vi "SL Basic Interface.vi"() -> ()   [LabVIEW 2016]
uses:
  source code/LSL components/scripts/scripts manager/scripts manager.lvclass
  source code/LSL components/output terminal/SystemLink OT/SystemLinkOutputTerminal.lvclass
  E:/Repository/LabVIEW Script Language/source code/LSL components/output terminal/Plain OT/PainOutputTerminal.lvclass
  E:/Repository/LabVIEW Script Language/source code/LSL components/output terminal/Base/Output Terminal.lvclass
  source code/LSL components/output terminal/Plain OT/PainOutputTerminal.lvclass/PainOutputTerminal.ctl
  source code/LSL components/output terminal/SystemLink OT/SystemLinkOutputTerminal.lvclass/SystemLinkOutputTerminal.ctl
  source code/LSL components/variables/RT Variables/RT Variables.lvclass
  source code/LSL components/scripts/scripts manager/scripts manager.lvclass/scripts manager.ctl
  <vilib>/Skyline/Message/AMQP/NI Skyline Message AMQP (Async).lvclass
  source code/LSL components/output terminal/Plain OT/properties/Write Output Terminal.vi
  source code/LSL components/output terminal/SystemLink OT/properties/Write SL async ref.vi
  source code/LSL components/output terminal/SystemLink OT/properties/Write Publish Topic.vi
  source code/LSL components/scripts/scripts manager/properties/Write Scripts.vi
  <vilib>/Skyline/Message/AMQP/async/Open (Async).vi
  <vilib>/Skyline/Utilities/NI Skyline Utilities.lvlib
  <vilib>/Skyline/Message/NI Skyline Message.lvclass
panel:
  in  "Help":bool
  in  "Script Compile":bool
  in  "Script Save":bool
  in  "Script Delete":bool
  in  "Script New":bool
  in  "Script Run":bool
  in  "Script Files":i32(listbox)
  out "Output Terminal":string
  in  "scripting pane":T1
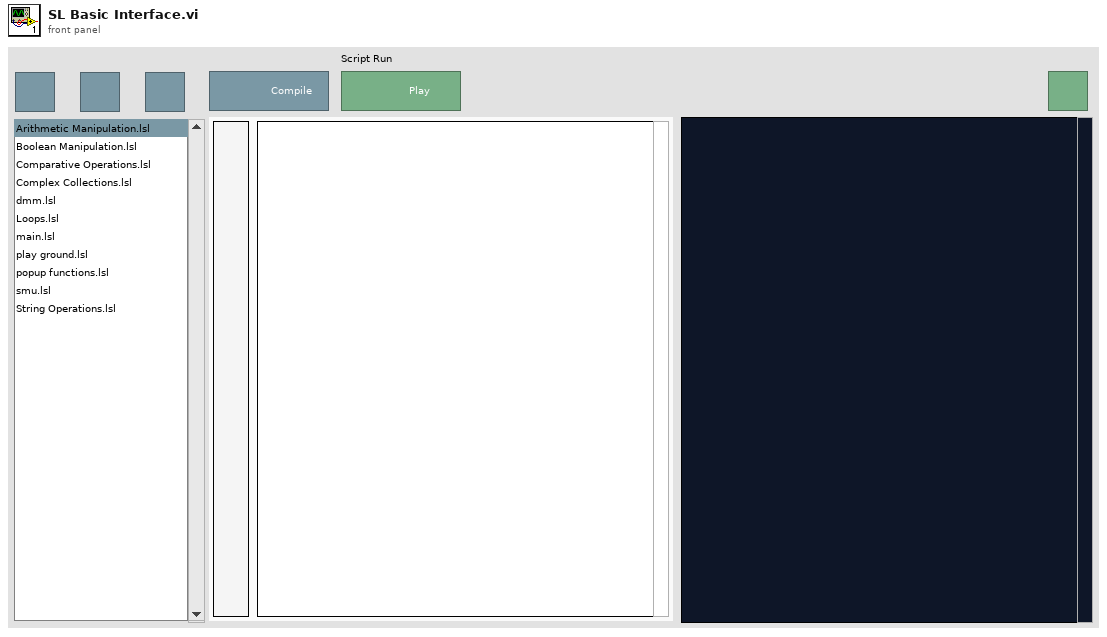
[diagram p1: front panel]
types:
  T1 = cluster{"Script Editor":string, "Script Editor":string}
  T2 = enum32{"Invalid", "Standard", "Closed", "Hidden", "Minimized", "Maximized"}
  T3 = enum32{"invalid app kind", "Development System", "Run Time System", "Student Edition", "Embedded LabVIEW", "Evaluation", "Custom"}
  T4 = cluster{"Core":cluster{"Current VI Reference":refnum<vi>, "Close Panel on Exit?":bool}, "scripts manager":refnum<class "scripts manager.lvclass">, "Script":string, "Config Folder":path, "SystemLink OT":refnum<class "SystemLinkOutputTerminal.lvclass">, "message async":refnum<class "NI Skyline Message AMQP (Async).lvclass">, "topic":string}
  T5 = cluster{"Current VI Reference":refnum<vi>, "Close Panel on Exit?":bool}
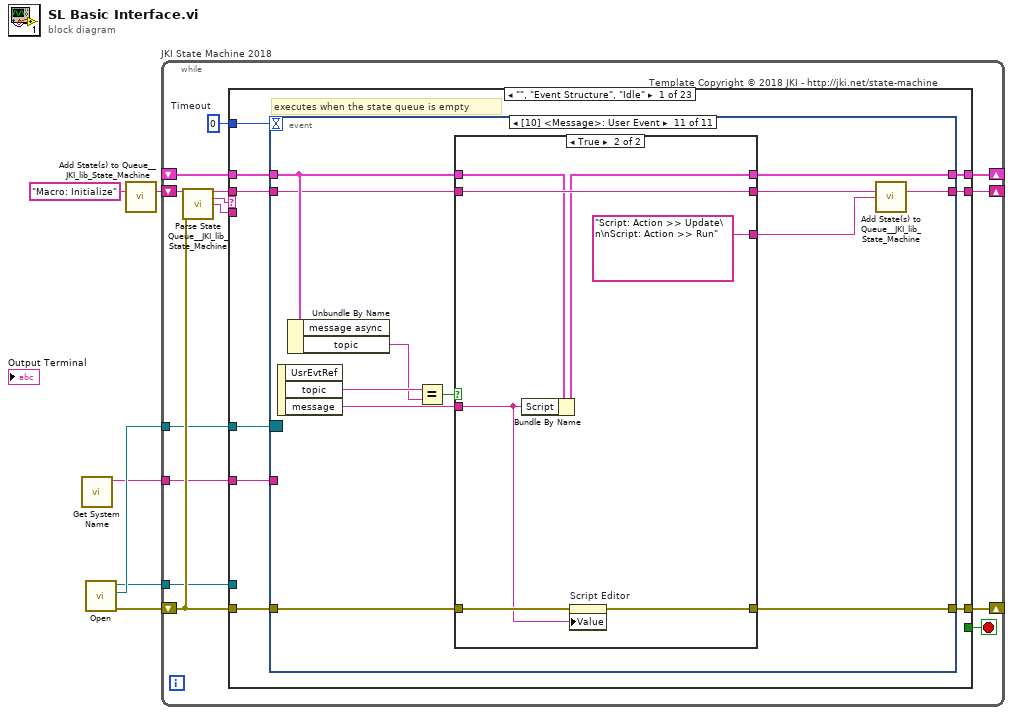
[diagram p0: block diagram]
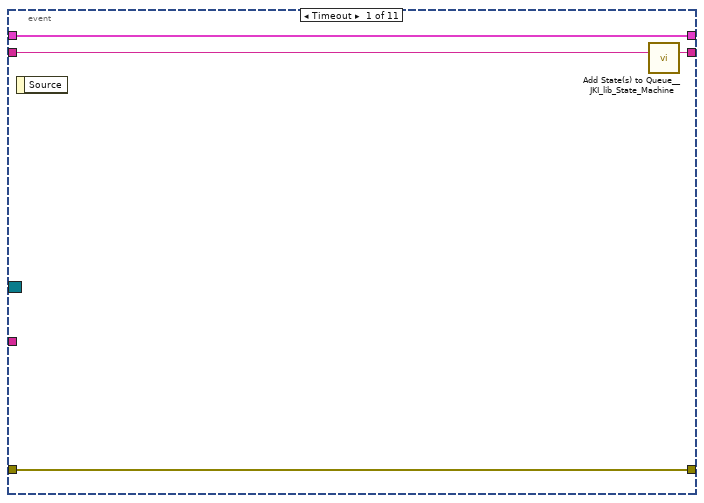
[diagram p2: hidden frame]
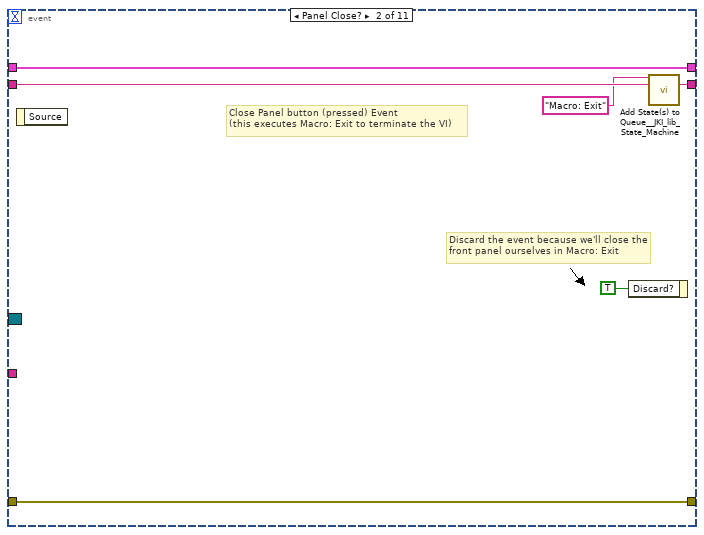
[diagram p3: hidden frame]
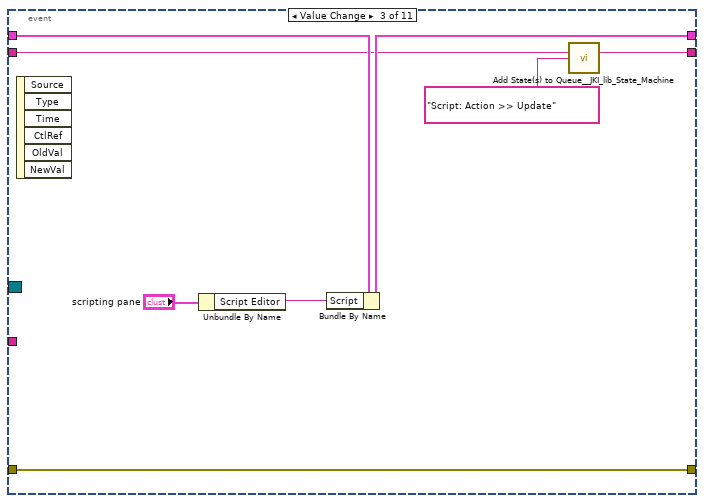
[diagram p4: hidden frame]
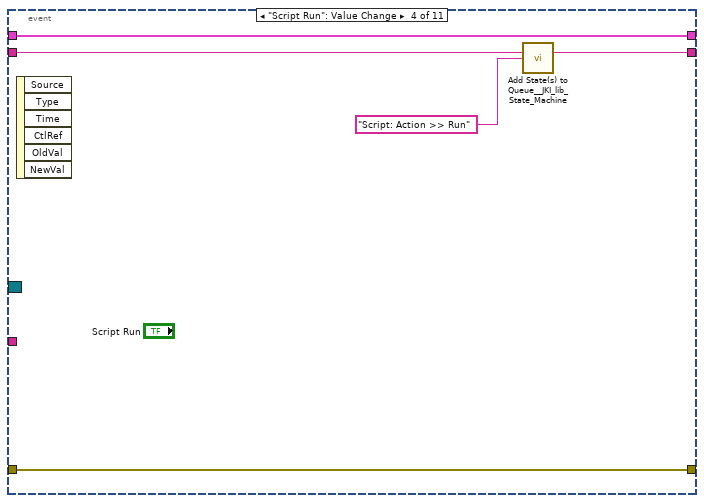
[diagram p5: hidden frame]
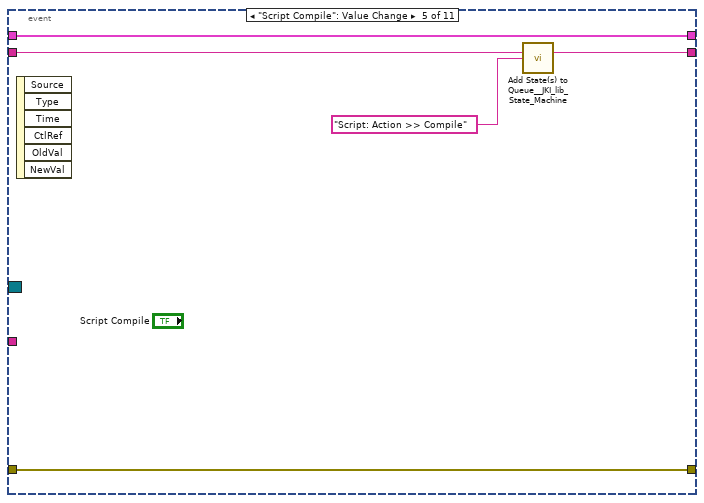
[diagram p6: hidden frame]
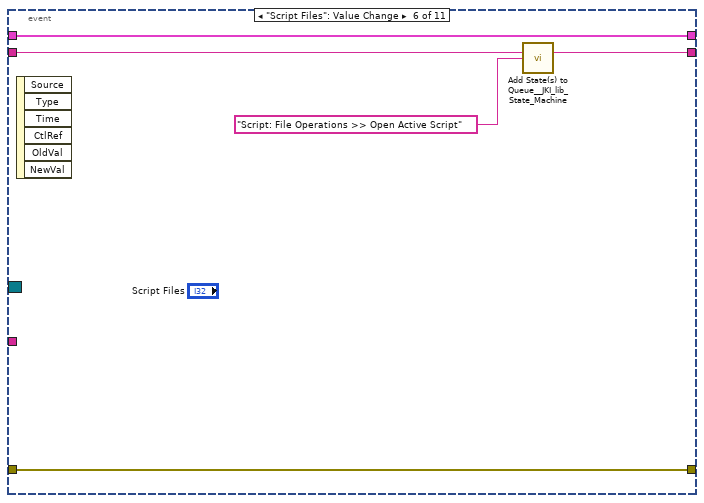
[diagram p7: hidden frame]
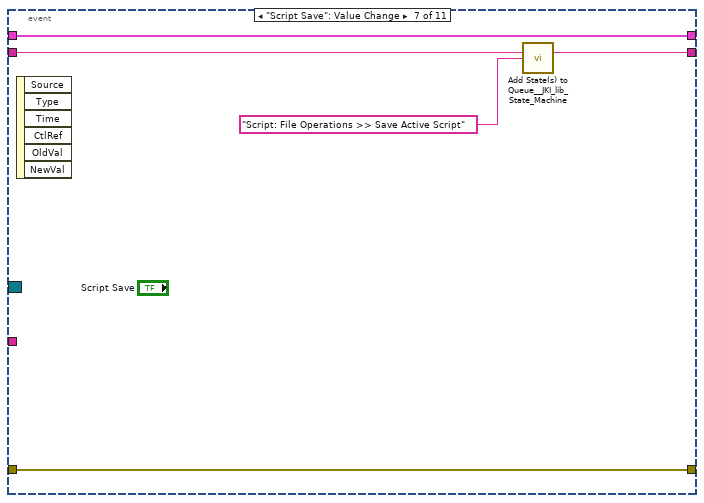
[diagram p8: hidden frame]
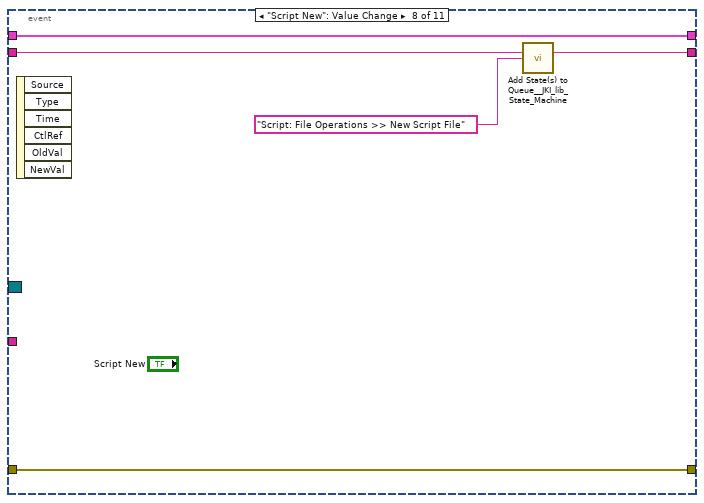
[diagram p9: hidden frame]
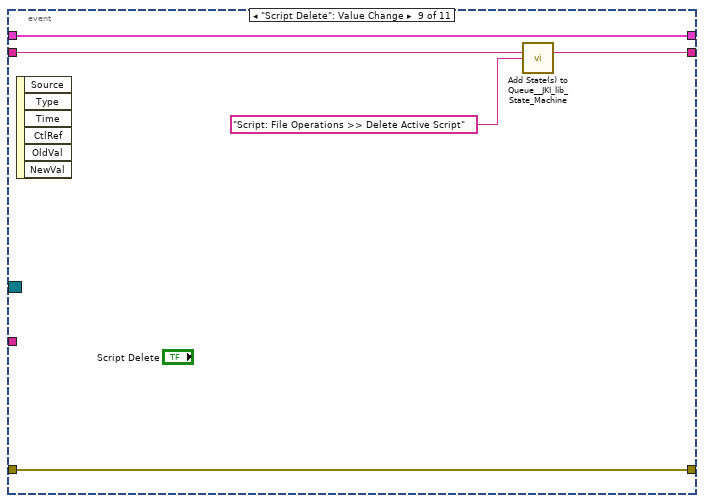
[diagram p10: hidden frame]
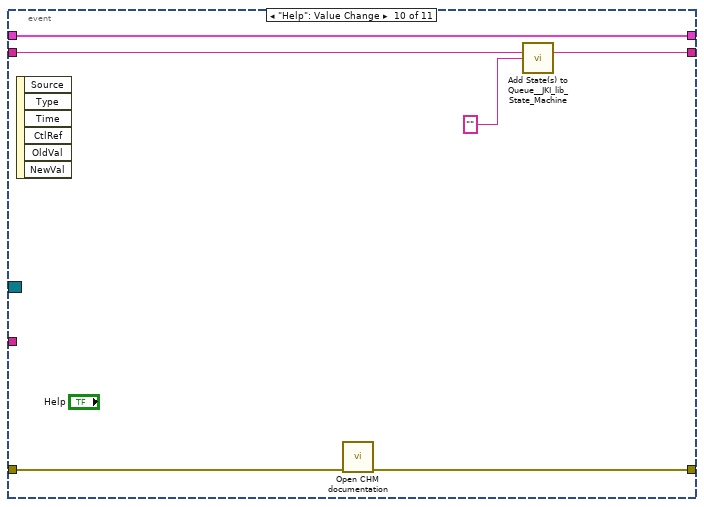
[diagram p11: hidden frame]
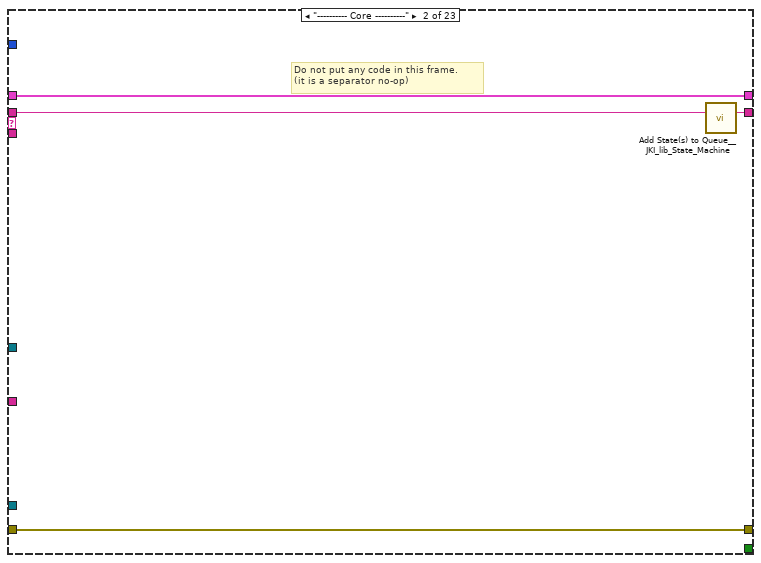
[diagram p13: hidden frame]
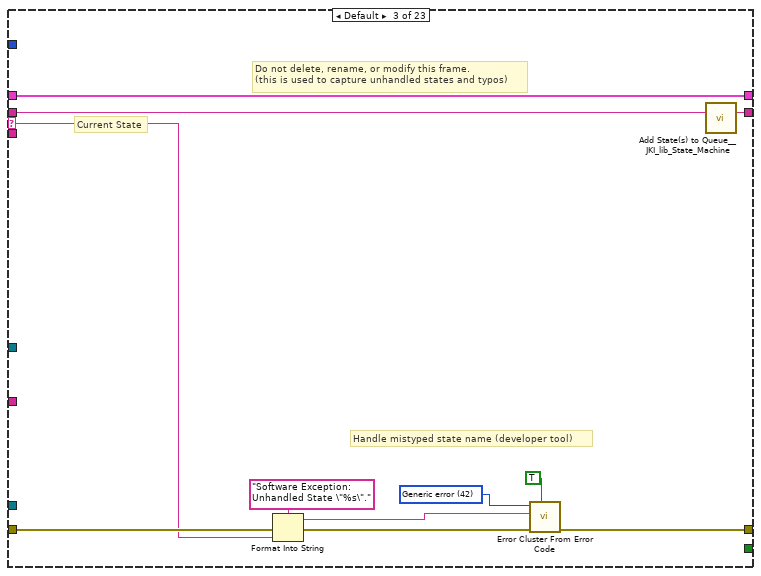
[diagram p14: hidden frame]
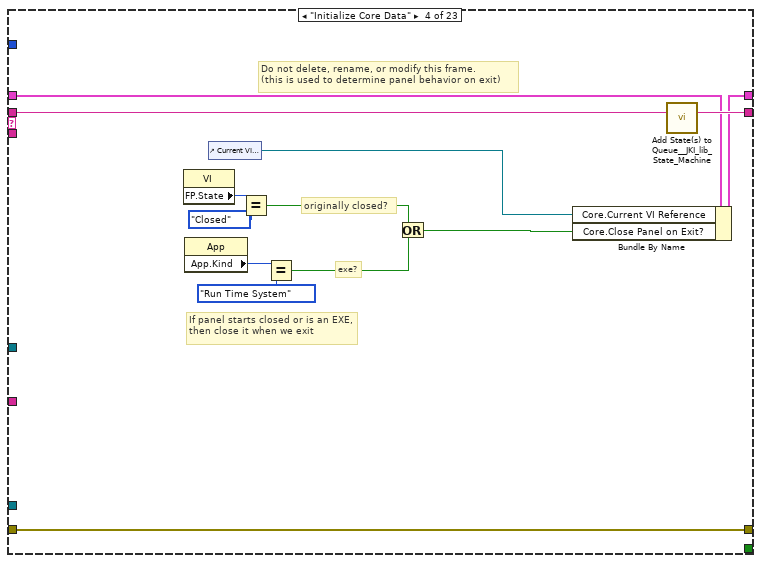
[diagram p15: hidden frame]
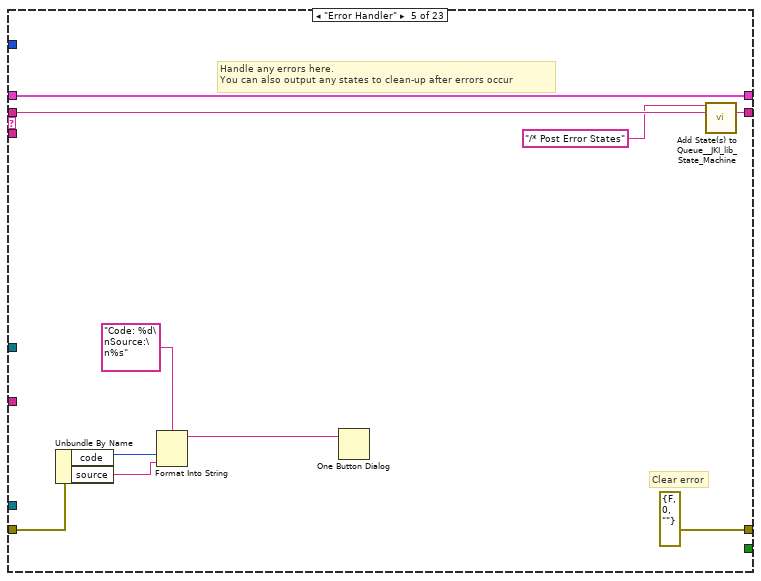
[diagram p16: hidden frame]
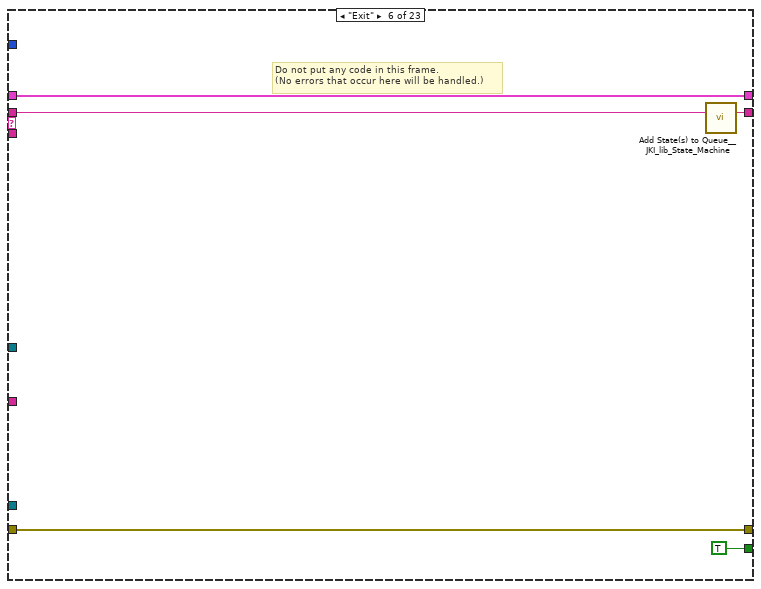
[diagram p17: hidden frame]
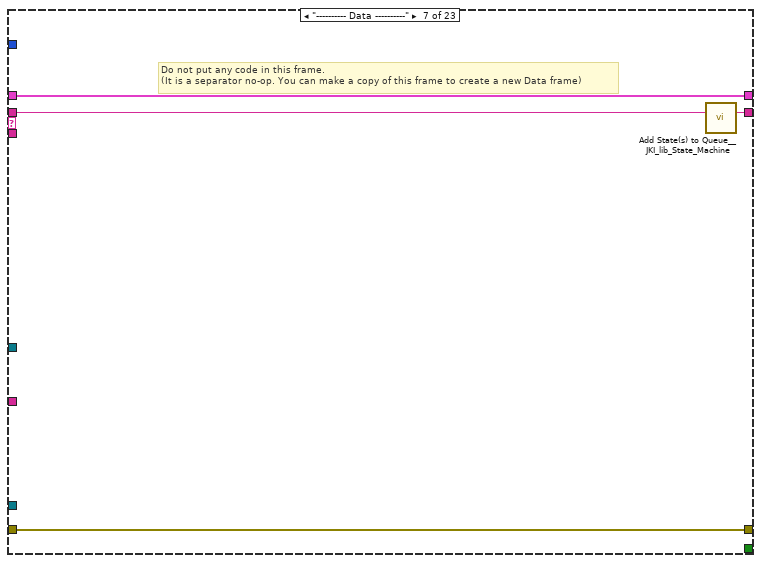
[diagram p18: hidden frame]
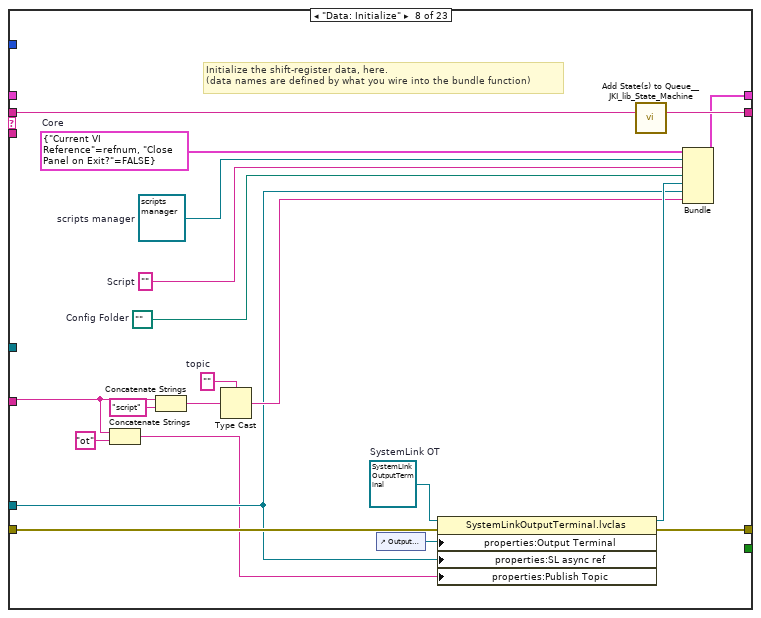
[diagram p19: hidden frame]
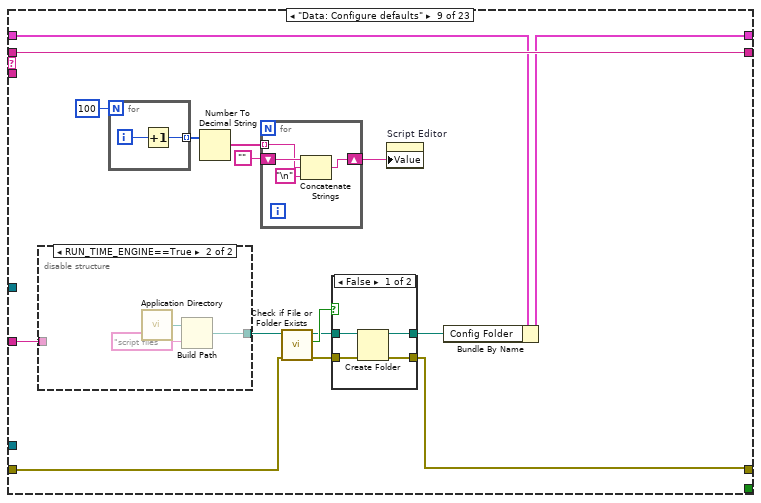
[diagram p20: hidden frame]
diagram:
  n1 = call <vilib>:"Get System Name.vi"() -> ("system name"=w1:string)  [unwired: 11 in]
  n2 = call-poly <vilib>:"Open.vi"() -> ("error out"=w3:errorcluster, "event registration reference"=w4:refnum<event-registration>, "message async"=w2:refnum<class "NI Skyline Message AMQP (Async).lvclass">)  [unwired: 9 in]
  n3 = call <vilib>:"Add State(s) to Queue__JKI_lib_State_Machine.vi"("State(s) in (\"\")"="Macro: Initialize") -> ("States Out"=w6:string)  [unwired: 14 in]
  n4 = while "JKI State Machine 2018" {
    shift-right: [w13] -> _
    shift-left: _ -> [w12]
    shift-right: [w16] -> _
    shift-left: w3 -> [w10]
    shift-right: [w15] -> _
    shift-left: w6 -> [w17]
    tunnel: w1 -> [w9]
    tunnel: w2 -> [w7]
    tunnel: w4 -> [w8]
    stop <- w14 stop-if-true
    w11 = 0  # Timeout
    # "Template Copyright © 2018 JKI - http://jki.net/state-machine"
    n5 = call <vilib>:"Parse State Queue__JKI_lib_State_Machine.vi"("State Queue"=w17, "Error In (no error)"=w10) -> ("Remaining States"=w19:string, "Current State"=w20:string, "Arguments"=w18:string)  [unwired: 11 in]
    n6 = case shown="\"\", \"Event Structure\", \"Idle\"" w20 {
      selector: w20 -> [_ _ w110 _ _ _ _ _ _ _ _ _ _ _ _ _ _ _ _ _ _ _ _]
      tunnel: w19 -> [w29 w109 w114 w133 w143 w148 w152 w172 w188 w214 w218 w230 w236 w247 w316 w321 w331 w335 w346 w376 w447 w456 w466]
      tunnel: w18 -> [_ _ _ _ _ _ _ _ _ _ _ _ w231 w241 _ _ _ _ w344 w384 _ _ _]
      tunnel: w12 -> [w27 w106 w112 w126 w140 w146 w149 _ w181 w209 w215 w228 w234 w243 w313 w318 w328 w332 w339 w383 w448 w451 w463]
      tunnel: [w26 w107 w116 w130 errorcluster {"status"=FALSE, "code"=0, "source"=""} ("error out") w145 w150 w164 w183 w210 w216 w225 w232 w244 w314 w319 w329 w333 w342 w385 w446 w454 w459] -> w16
      tunnel: w10 -> [w25 w107 w115 w130 w138 w145 w150 w165 w184 w211 w216 w226 w233 w245 w314 w319 w329 w333 w343 w380 w446 w455 w465]
      tunnel: [w28 w108 w113 w132 w142 w147 w151 w171 w188 w213 w217 w229 w235 w246 w315 w320 w330 w334 w345 w377 w447 w456 w466] -> w15
      tunnel: [_ _ _ _ _ TRUE _ _ _ _ _ _ _ _ _ _ _ _ _ _ _ _ _] -> w14
      tunnel: [w24 w106 w112 w131 w140 w146 w149 w169 w180 w209 w215 w228 w234 w243 w313 w318 w328 w332 w338 w383 w448 w450 w462] -> w13
      tunnel: w11 -> [w23 _ _ _ _ _ _ _ _ _ _ _ _ _ _ _ _ _ _ _ _ _ _]
      tunnel: w9 -> [w21 _ _ _ _ _ _ w155 w173 _ _ _ _ _ _ _ _ _ _ _ _ _ _]
      tunnel: w8 -> [w22 _ _ _ _ _ _ _ _ _ _ _ _ _ _ _ _ _ _ _ _ _ _]
      tunnel: w7 -> [_ _ _ _ _ _ _ w156 _ _ _ _ _ _ _ _ _ _ _ _ _ _ _]
      frame "", "Event Structure", "Idle" {
        # "executes when the state queue is empty"
        n7 = event shown="[10] <Message>: User Event" {
          selector: w22 -> [_ _ _ _ _ _ _ _ _ _ _]
          dyn-events: _ -> [_ _ _ _ _ _ _ _ _ _ _]
          timeout: w23 -> [_ _ _ _ _ _ _ _ _ _ _]
          tunnel: w29 -> [w33 w39 w42 w49 w54 w59 w64 w69 w74 w81 w87]
          tunnel: [w32 w38 w43 w50 w55 w60 w65 w70 w75 w82 w86] -> w28
          tunnel: w27 -> [w30 w36 w45 w52 w57 w62 w67 w72 w77 w83 w89]
          tunnel: [w31 w37 w40 w51 w56 w61 w66 w71 w76 w78 w85] -> w26
          tunnel: w25 -> [w31 w37 w40 w51 w56 w61 w66 w71 w76 w79 w92]
          tunnel: [w30 w36 w44 w52 w57 w62 w67 w72 w77 w83 w90] -> w24
          tunnel: w21 -> [_ _ _ _ _ _ _ _ _ _ _]
          event Timeout {
            n8 = event-data() -> ()  [unwired: 1 in, 1 out]
            n9 = call <vilib>:"Add State(s) to Queue__JKI_lib_State_Machine.vi"("State(s) in (\"\")"=w33) -> ("States Out"=w32:string)  [unwired: 14 in]
          }
          event Panel Close? {
            # "Discard the event because we'll close the front panel ourselves in Macro: Exit"
            # "Close Panel button (pressed) Event\n(this executes Macro: Exit to terminate the VI)"
            n10 = event-data() -> ()  [unwired: 1 in, 1 out]
            n11 = event-data("Discard?"=TRUE) -> ()  [unwired: 1 in, 1 out]
            n12 = call <vilib>:"Add State(s) to Queue__JKI_lib_State_Machine.vi"("State(s) in Front (\"\")"="Macro: Exit", "State(s) in (\"\")"=w39) -> ("States Out"=w38:string)  [unwired: 13 in]
          }
          event "scripting pane.Script Editor": Value Change {
            n13 = event-data() -> ()  [unwired: 1 in, 6 out]
            n14 = Unbundle By Name("scripting pane") -> ("Script Editor"=w46:string)
            n15 = Bundle By Name(cluster=w45, "Script"=w46) -> (w44:T4)
            n16 = call <vilib>:"Add State(s) to Queue__JKI_lib_State_Machine.vi"("State(s) in (\"\")"=w42, "State(s) at Back (\"\")"="Script: Action >> Update" ("State(s) at Back (\"\")")) -> ("States Out"=w43:string)  [unwired: 13 in]
          }
          event "Script Run": Value Change {
            n17 = event-data() -> ()  [unwired: 1 in, 6 out]
            n18 = call <vilib>:"Add State(s) to Queue__JKI_lib_State_Machine.vi"("State(s) in (\"\")"=w49, "State(s) at Back (\"\")"="Script: Action >> Run" ("State(s) at Back (\"\")")) -> ("States Out"=w50:string)  [unwired: 13 in]
          }
          event "Script Compile": Value Change {
            n19 = event-data() -> ()  [unwired: 1 in, 6 out]
            n20 = call <vilib>:"Add State(s) to Queue__JKI_lib_State_Machine.vi"("State(s) in (\"\")"=w54, "State(s) at Back (\"\")"="Script: Action >> Compile" ("State(s) at Back (\"\")")) -> ("States Out"=w55:string)  [unwired: 13 in]
          }
          event "Script Files": Value Change {
            n21 = event-data() -> ()  [unwired: 1 in, 6 out]
            n22 = call <vilib>:"Add State(s) to Queue__JKI_lib_State_Machine.vi"("State(s) in (\"\")"=w59, "State(s) at Back (\"\")"="Script: File Operations >> Open Active Script" ("State(s) at Back (\"\")")) -> ("States Out"=w60:string)  [unwired: 13 in]
          }
          event "Script Save": Value Change {
            n23 = event-data() -> ()  [unwired: 1 in, 6 out]
            n24 = call <vilib>:"Add State(s) to Queue__JKI_lib_State_Machine.vi"("State(s) in (\"\")"=w64, "State(s) at Back (\"\")"="Script: File Operations >> Save Active Script" ("State(s) at Back (\"\")")) -> ("States Out"=w65:string)  [unwired: 13 in]
          }
          event "Script New": Value Change {
            n25 = event-data() -> ()  [unwired: 1 in, 6 out]
            n26 = call <vilib>:"Add State(s) to Queue__JKI_lib_State_Machine.vi"("State(s) in (\"\")"=w69, "State(s) at Back (\"\")"="Script: File Operations >> New Script File" ("State(s) at Back (\"\")")) -> ("States Out"=w70:string)  [unwired: 13 in]
          }
          event "Script Delete": Value Change {
            n27 = event-data() -> ()  [unwired: 1 in, 6 out]
            n28 = call <vilib>:"Add State(s) to Queue__JKI_lib_State_Machine.vi"("State(s) in (\"\")"=w74, "State(s) at Back (\"\")"="Script: File Operations >> Delete Active Script" ("State(s) at Back (\"\")")) -> ("States Out"=w75:string)  [unwired: 13 in]
          }
          event "Help": Value Change {
            n29 = event-data() -> ()  [unwired: 1 in, 6 out]
            n30 = call "Open CHM documentation.vi"("error in"=w79) -> ("error out"=w78:errorcluster)  [unwired: 10 in]
            n31 = call <vilib>:"Add State(s) to Queue__JKI_lib_State_Machine.vi"("State(s) in (\"\")"=w81, "State(s) at Back (\"\")"="" ("State(s) at Back (\"\")")) -> ("States Out"=w82:string)  [unwired: 13 in]
          }
          event User Event {
            n32 = event-data() -> ("topic"=w95:string, "message"=w91:string)  [unwired: 1 in, 1 out]
            n33 = Unbundle By Name(w89) -> ("topic"=w94:string)  [unwired: 1 out]
            n34 = Equal?(x=w95, y=w94) -> (x = y?=w93:bool)
            n35 = case shown="True" w93 {
              tunnel: w92 -> [w96 w101]
              tunnel: w91 -> [_ w99]
              tunnel: [w98 w102] -> w90
              tunnel: w89 -> [w98 w103]
              tunnel: [w97 w105] -> w88
              tunnel: w87 -> [w97 w105]
              tunnel: [w96 w100] -> w85
              tunnel: [_ "Script: Action >> Update\n\nScript: Action >> Run" ("State(s) at Back (\"\")")] -> w84
              frame False {
              }
              frame True {
                n36 = Bundle By Name(cluster=w103, "Script"=w99) -> (w102:T4)
                n37 = property on="Script Editor" class="Str"(error in=w101, "Value"=w99) -> (error out=w100:errorcluster)  [unwired: 1 in, 1 out]
              }
            }
            n38 = call <vilib>:"Add State(s) to Queue__JKI_lib_State_Machine.vi"("State(s) in (\"\")"=w88, "State(s) at Back (\"\")"=w84) -> ("States Out"=w86:string)  [unwired: 13 in]
          }
        }
      }
      frame "---------- Core ----------" {
        # "Do not put any code in this frame.\n(it is a separator no-op)"
        n39 = call <vilib>:"Add State(s) to Queue__JKI_lib_State_Machine.vi"("State(s) in (\"\")"=w109) -> ("States Out"=w108:string)  [unwired: 14 in]
      }
      frame Default {
        w119 = 42 items=["No error", "Argument error", "Memory is full", "Out of zone", "End of file", "File already open", "Generic file I/O error", "File not found", "File permission error", "Disk is full", "Duplicate path", "Too many files open", "System feature not enabled", "Resource file not found", "Cannot add resource", "Resource not found", "Image not found", "Image memory error", "Pen does not exist", "Config type invalid", "Config token not found", "Config parse error", "Config memory error", "Bad external code format", "Bad external code offset", "External code not present", "Null window", "Destroy window error", "Null menu", "Print aborted", "Bad print record", "Print driver error", "Windows error during printing", "Memory error during printing", "Print dialog error", "Generic print error", "Invalid device refnum", "Device not found", "Device parameter error", "Device unit error", "Cannot open device", "Device call aborted", "Generic error", "Cancelled by user", "Object ID too low", "Object ID too high", "Object not in heap", "Unknown heap", "Unknown object (invalid DefProc)", "Unknown object (DefProc not in table)", "Message out of range", "Invalid (null) method", "Unknown message", "Manager call not supported", "Bad address", "Network operation in progress", "Network operation timed out", "Connection is busy", "Network attribute not supported", "Network error", "Address in use", "System out of memory", "Connection aborted", "Connection refused", "Not connected", "Already connected", "Connection closed", "Initialization error (interapplication manager)", "Bad occurrence", "Wait on unbound occurrence handler", "Occurrence queue overflow", "Datalog type conflict", "Unused", "Unrecognized type (interapplication manager)", "Memory corrupt", "Failed to make temporary DLL", "Old CIN version", "Drag socket not found", "Failed to load drop-object", "Failed to register OLE object", "Failed to release OLE object", "Format specifier type mismatch", "Unknown format specifier", "Too few format specifiers", "Too many format specifiers", "Scan failed", "Newer CIN version", "Error converting to variant", "Runtime menu error", "Password tampered", "Variant attribute not found", "Incompatible variant data type", "Event data is not available", "Event Store is not present", "Occurrence is not found", "Event Queue is not created", "Event info is not available", "Refnum passed is NULL", "Error retrieving Class GUID", "Error retrieving CoClass GUID", "Error retrieving TypeLib GUID.", "Bad built application magic bytes.", "Specific driver is different from the specific driver associated with the Logical Name.", "There is no session opened to the class driver.", "Max Error", "MAX - Error with config objects", "MAX - Error loading configuration", "MAX - Group not supported"]
        # "Current State"
        # "Do not delete, rename, or modify this frame.\n(this is used to capture unhandled states and typos)"
        # "Handle mistyped state name (developer tool)"
        n40 = Format Into String(format string="Software Exception: Unhandled State \"%s\"." ("message"), error in=w115, w110) -> (resulting string=w118:string, error out=w117:errorcluster)  [unwired: 1 in]
        n41 = call <vilib>:"Error Cluster From Error Code.vi"("show call chain? (False)"=TRUE, "error in (no error)"=w117, "error message (\"\")"=w118, "error code (0)"=w119) -> ("error out"=w116:errorcluster)  [unwired: 5 in]
        n42 = call <vilib>:"Add State(s) to Queue__JKI_lib_State_Machine.vi"("State(s) in (\"\")"=w114) -> ("States Out"=w113:string)  [unwired: 14 in]
      }
      frame "Initialize Core Data" {
        # "Do not delete, rename, or modify this frame.\n(this is used to determine panel behavior on exit)"
        # "originally closed?"
        # "exe?"
        # "If panel starts closed or is an EXE, then close it when we exit"
        n43 = property class="VI"() -> ("FP.State"=w123:T2)  [unwired: 2 in, 2 out]
        n44 = property class="App"() -> ("App.Kind"=w129:T3)  [unwired: 2 in, 2 out]
        n45 = control-ref of="Current VI Reference"() -> (w124:refnum<vi>)
        n46 = Equal?(x=w123, y=T2."Closed" ("Front Panel Window:State")) -> (x = y?=w121:bool)
        n47 = Equal?(x=w129, y=T3."Run Time System" ("Application:Kind")) -> (x = y?=w127:bool)
        n48 = Or(x=w121, y=w127) -> (x .or. y?=w125:bool)
        n49 = Bundle By Name(cluster=w126, "Core.Current VI Reference"=w124, "Core.Close Panel on Exit?"=w125) -> (w131:T4)
        n50 = call <vilib>:"Add State(s) to Queue__JKI_lib_State_Machine.vi"("State(s) in (\"\")"=w133) -> ("States Out"=w132:string)  [unwired: 14 in]
      }
      frame "Error Handler" {
        # "Handle any errors here.\nYou can also output any states to clean-up after errors occur"
        # "Clear error"
        n51 = Unbundle By Name(w138) -> ("code"=w137:i32, "source"=w136:string)
        n52 = Format Into String(format string="Code: %d\nSource:\n%s", w137, w136) -> (resulting string=w134:string)  [unwired: 2 in, 1 out]
        n53 = One Button Dialog(message=w134) -> ()  [unwired: 1 in, 1 out]
        n54 = call <vilib>:"Add State(s) to Queue__JKI_lib_State_Machine.vi"("State(s) in Front (\"\")"="/* Post Error States", "State(s) in (\"\")"=w143) -> ("States Out"=w142:string)  [unwired: 13 in]
      }
      frame "Exit" {
        # "Do not put any code in this frame.\n(No errors that occur here will be handled.)"
        n55 = call <vilib>:"Add State(s) to Queue__JKI_lib_State_Machine.vi"("State(s) in (\"\")"=w148) -> ("States Out"=w147:string)  [unwired: 14 in]
      }
      frame "---------- Data ----------" {
        # "Do not put any code in this frame.\n(It is a separator no-op. You can make a copy of this frame to create a new Data frame)"
        n56 = call <vilib>:"Add State(s) to Queue__JKI_lib_State_Machine.vi"("State(s) in (\"\")"=w152) -> ("States Out"=w151:string)  [unwired: 14 in]
      }
      frame "Data: Initialize" {
        w157 = refnum<class "SystemLinkOutputTerminal.lvclass"> refnum  # SystemLink OT
        w160 = ""  # topic
        w162 = path ""  # Config Folder
        w167 = ""  # Script
        w168 = refnum<class "scripts manager.lvclass"> refnum  # scripts manager
        w170 = T5 {"Current VI Reference"=refnum, "Close Panel on Exit?"=FALSE}  # Core
        # "Initialize the shift-register data, here.\n(data names are defined by what you wire into the bundle function)"
        n57 = Concatenate Strings(w155, "ot" ("string")) -> (w153:string)
        n58 = Concatenate Strings(w155, "script" ("string")) -> (w159:string)
        n59 = Type Cast(type=w160, x=w159) -> (*(type *) &x=w158:string)
        n60 = control-ref of="Output Terminal"() -> (w163:refnum<vi>)
        n61 = property class="SystemLinkOutputTerminal.lvclas"(reference=w157, error in=w165, "properties:Output Terminal"=w163, "properties:SL async ref"=w156, "properties:Publish Topic"=w153) -> (reference out=w166:refnum<class "SystemLinkOutputTerminal.lvclass">, error out=w164:errorcluster)
        n62 = call <vilib>:"Add State(s) to Queue__JKI_lib_State_Machine.vi"("State(s) in (\"\")"=w172) -> ("States Out"=w171:string)  [unwired: 14 in]
        n63 = Bundle("Core"=w170, "scripts manager"=w168, "Script"=w167, "Config Folder"=w162, "SystemLink OT"=w166, "message async"=w156, "topic"=w158) -> (w169:T4)  [unwired: 1 in]
      }
      frame "Data: Configure defaults" {
        n64 = disable-structure shown="RUN_TIME_ENGINE==True" {
          disable-tunnel: [w190 w194] -> w174
          disable-tunnel: w173 -> [w189 _]
          frame condition #0 (active) {
            n65 = call <vilib>:"Application Directory.vi"() -> ("Application Directory"=w192:path)
            n66 = Build Path(base path=w192, name or relative path="example") -> (appended path=w191:path)
            n67 = Build Path(base path=w191, name or relative path=w189) -> (appended path=w190:path)
          }
          frame condition #1 {
            n68 = call <vilib>:"Application Directory.vi"() -> ("Application Directory"=w195:path)
            n69 = Build Path(base path=w195, name or relative path="script files") -> (appended path=w194:path)
          }
        }
        n70 = for {
          N: 100 -> [_]
          tunnel: [w201] -> w178 mode=indexing
          i -> [w202]
          n71 = Increment(x=w202) -> (x+1=w201:i32)
        }
        n72 = Number To Decimal String(number=w178) -> (decimal integer string=w176:string[])  [unwired: 1 in]
        n73 = for {
          tunnel: w176 -> [w197] mode=indexing
          shift-right: [w200] -> w177
          shift-left: "" -> [w198]
          n74 = Concatenate Strings(w198, w197, "\n") -> (w200:string)
        }
        n75 = call <vilib>:"Check if File or Folder Exists.vi"("error in (no error)"=w184, "path"=w174) -> ("error out"=w185:errorcluster, "file or folder exists?"=w187:bool, "dup path"=w186:path)  [unwired: 7 in]
        n76 = case shown="False" w187 {
          tunnel: w185 -> [w206 w207]
          tunnel: w186 -> [w205 w208]
          tunnel: [w203 w208] -> w182
          tunnel: [w204 w207] -> w183
          frame False {
            n77 = Create Folder(path (use dialog)=w205, error in=w206) -> (created path=w203:path, error out=w204:errorcluster)  [unwired: 1 in, 1 out]
          }
          frame True {
          }
        }
        n78 = property on="Script Editor" class="Str"("Value"=w177) -> ()  [unwired: 2 in, 2 out]
        n79 = Bundle By Name(cluster=w181, "Config Folder"=w182) -> (w180:T4)
      }
      frame "Data: Cleanup" {
        # "Cleanup any data and references, here.\n(this is called automatically, by the Macro: Exit)"
        n80 = Unbundle By Name(w209) -> ("Core.Current VI Reference"=w212:refnum<vi>)
        n81 = Close Reference(reference=w212, error in (no error)=w211) -> (error out=w210:errorcluster)
        n82 = call <vilib>:"Add State(s) to Queue__JKI_lib_State_Machine.vi"("State(s) in (\"\")"=w214) -> ("States Out"=w213:string)  [unwired: 14 in]
      }
      frame "---------- UI ----------" {
        # "Do not put any code in this frame.\n(It is a separator no-op. You can make a copy of this frame to create a new UI frame)"
        n83 = call <vilib>:"Add State(s) to Queue__JKI_lib_State_Machine.vi"("State(s) in (\"\")"=w218) -> ("States Out"=w217:string)  [unwired: 14 in]
      }
      frame "UI: Initialize" {
        w223 = u32 923176
        # "Initialize the User Interface, here.\n(this is called automatically, by the Macro: Init)"
        n84 = property on="Script Editor" class="Str"("Text.BG Color"=u32 16119285) -> ()  [unwired: 2 in, 2 out]
        n85 = property on="Output Terminal" class="Str"("Text.BG Color"=w223, "Text.BGColor"=w223, "Text.TextColor"=u32 16777215) -> ()  [unwired: 2 in, 2 out]
        n86 = property on="Script Files" class="LstBox (strict)"("Item Names"=string[] []) -> ()  [unwired: 2 in, 2 out]
        n87 = property on="Script Files" class="LstBox (strict)"(error in=w226, "SelColor"=u32 8034469) -> (error out=w225:errorcluster)  [unwired: 1 in, 1 out]
        n88 = local write "Output Terminal"("" ("Output Terminal")) -> ()
        n89 = local write "scripting pane"(T1 {"Script Editor"="", "Script Editor"=""} ("scripting pane")) -> ()
        n90 = call <vilib>:"Add State(s) to Queue__JKI_lib_State_Machine.vi"("State(s) in (\"\")"=w230) -> ("States Out"=w229:string)  [unwired: 14 in]
      }
      frame "UI: Cursor Set" {
        # "Argument"
        # "Set and Unset Cursor Busy.\n(Usage: \"UI: Cursor Set >> Busy|Idle\")"
        n91 = case shown="\"Idle\", Default" w231 {
          tunnel: w233 -> [w238 w240]
          tunnel: [w237 w239] -> w232
          frame "Idle", Default {
            n92 = call <vilib>:"Unset Busy.vi"("error in (no error)"=w238) -> ("error out"=w237:errorcluster)  [unwired: 10 in]
          }
          frame "Busy" {
            n93 = call <vilib>:"Set Busy.vi"("error in (no error)"=w240) -> ("error out"=w239:errorcluster)  [unwired: 9 in, 1 out]
          }
        }
        n94 = call <vilib>:"Add State(s) to Queue__JKI_lib_State_Machine.vi"("State(s) in (\"\")"=w236) -> ("States Out"=w235:string)  [unwired: 14 in]
      }
      frame "UI: Front Panel State" {
        # "Argument"
        # "Set Front Panel Open or Closed\n(Usage: \"UI: Front Panel State >> Open|Close\")"
        n95 = Unbundle By Name(w243) -> ("Core.Current VI Reference"=w242:refnum<vi>)
        n96 = case shown="\"Minimize\", \"Minimized\"" w241 {
          tunnel: w245 -> [w253 w268 w279 w292 w305]
          tunnel: [w255 w269 w281 w294 w307] -> w244
          tunnel: w242 -> [w254 w266 w280 w293 w306]
          frame "Open", "Standard", Default {
            w248 = T2."Standard" ("State")
            n97 = property class="VI"(reference=w254, error in=w253) -> (reference out=w251:refnum<vi>, error out=w252:errorcluster, "FP.State"=w250:T2)
            n98 = Not Equal?(x=w250, y=w248) -> (x != y?=w249:bool)
            n99 = case shown="True" w249 {
              tunnel: [w259 w261] -> w255
              tunnel: w252 -> [w258 w261]
              tunnel: w251 -> [w257 _]
              tunnel: w248 -> [w256 _]
              frame True {
                n100 = invoke class="VI" method="FP.Open"(reference=w257, error in=w258, "Activate"=TRUE, "State"=w256) -> (error out=w259:errorcluster)  [unwired: 1 in, 4 out]
              }
              frame False {
              }
            }
          }
          frame "Close", "Closed" {
            n101 = property class="VI"(reference=w266, error in=w268) -> (reference out=w265:refnum<vi>, error out=w267:errorcluster, "FP.State"=w263:T2)
            n102 = Not Equal?(x=w263, y=T2."Closed" ("Front Panel Window:State")) -> (x != y?=w262:bool)
            n103 = case shown="True" w262 {
              tunnel: [w270 w273] -> w269
              tunnel: w267 -> [w270 w272]
              tunnel: w265 -> [_ w271]
              frame False {
              }
              frame True {
                n104 = invoke class="VI" method="FP.Close"(reference=w271, error in=w272) -> (error out=w273:errorcluster)  [unwired: 1 in, 2 out]
              }
            }
          }
          frame "Hidden", "Hide" {
            w274 = T2."Hidden" ("State")
            n105 = property class="VI"(reference=w280, error in=w279) -> (reference out=w277:refnum<vi>, error out=w278:errorcluster, "FP.State"=w276:T2)
            n106 = Not Equal?(x=w276, y=w274) -> (x != y?=w275:bool)
            n107 = case shown="True" w275 {
              tunnel: [w285 w286] -> w281
              tunnel: w278 -> [w284 w286]
              tunnel: w277 -> [w283 _]
              tunnel: w274 -> [w282 _]
              frame True {
                n108 = invoke class="VI" method="FP.Open"(reference=w283, error in=w284, "State"=w282) -> (error out=w285:errorcluster)  [unwired: 2 in, 4 out]
              }
              frame False {
              }
            }
          }
          frame "Minimize", "Minimized" {
            w287 = T2."Minimized" ("State")
            n109 = property class="VI"(reference=w293, error in=w292) -> (reference out=w290:refnum<vi>, error out=w291:errorcluster, "FP.State"=w289:T2)
            n110 = Not Equal?(x=w289, y=w287) -> (x != y?=w288:bool)
            n111 = case shown="True" w288 {
              tunnel: [w298 w299] -> w294
              tunnel: w291 -> [w297 w299]
              tunnel: w290 -> [w296 _]
              tunnel: w287 -> [w295 _]
              frame True {
                n112 = invoke class="VI" method="FP.Open"(reference=w296, error in=w297, "State"=w295) -> (error out=w298:errorcluster)  [unwired: 2 in, 4 out]
              }
              frame False {
              }
            }
          }
          frame "Maximize", "Maximized" {
            w300 = T2."Maximized" ("State")
            n113 = property class="VI"(reference=w306, error in=w305) -> (reference out=w303:refnum<vi>, error out=w304:errorcluster, "FP.State"=w302:T2)
            n114 = Not Equal?(x=w302, y=w300) -> (x != y?=w301:bool)
            n115 = case shown="True" w301 {
              tunnel: [w311 w312] -> w307
              tunnel: w304 -> [w310 w312]
              tunnel: w303 -> [w309 _]
              tunnel: w300 -> [w308 _]
              frame True {
                n116 = invoke class="VI" method="FP.Open"(reference=w309, error in=w310, "State"=w308) -> (error out=w311:errorcluster)  [unwired: 2 in, 4 out]
              }
              frame False {
              }
            }
          }
        }
        n117 = call <vilib>:"Add State(s) to Queue__JKI_lib_State_Machine.vi"("State(s) in (\"\")"=w247) -> ("States Out"=w246:string)  [unwired: 14 in]
      }
      frame "---------- Macro ----------" {
        # "Do not put any code in this frame.\n(It is a separator no-op. You can make a copy of this frame to create a new Macro frame)"
        n118 = call <vilib>:"Add State(s) to Queue__JKI_lib_State_Machine.vi"("State(s) in (\"\")"=w316) -> ("States Out"=w315:string)  [unwired: 14 in]
      }
      frame "Macro: Initialize" {
        w317 = "Data: Initialize\nInitialize Core Data\nUI: Initialize\nUI: Front Panel State >> Open\nData: Configure defaults\n\nSL: Subscribe\n\nScript: Action >> Init\nScript: File Operations >>List Script File\nScript: File Operations >> Open Active Script"  # Data: Initialize Initialize Core Data UI: Initialize UI: Front Panel State >> Open Data: Configure defaults  SL: Subscribe  Script: Action >> Init Script: File Operations >>List Script File Script: File Operations >> Open Active Script
        # "Initialization Macro\n(This is called once, when the VI starts)"
        n119 = call <vilib>:"Add State(s) to Queue__JKI_lib_State_Machine.vi"("State(s) in Front (\"\")"=w317, "State(s) in (\"\")"=w321) -> ("States Out"=w320:string)  [unwired: 13 in]
      }
      frame "Macro: Exit" {
        # "Exit Macro\n(This is called once, when the VI exits)"
        n120 = Unbundle By Name(w328) -> ("Core.Close Panel on Exit?"=w327:bool)
        n121 = Select(t="UI: Front Panel State >> Close", s=w327, f="") -> (s? t:f=w324:string)
        n122 = call <vilib>:"Add State(s) to Queue__JKI_lib_State_Machine.vi"("State(s) in (\"\")"=w324, "State(s) at Back (\"\")"="Data: Cleanup\n\nScript: Action >> Close\n\nSL: Unsubscribe & Close\n\nExit") -> ("States Out"=w322:string)  [unwired: 13 in]
        n123 = call <vilib>:"Add State(s) to Queue__JKI_lib_State_Machine.vi"("State(s) in Front (\"\")"=w322, "State(s) in (\"\")"=w331) -> ("States Out"=w330:string)  [unwired: 13 in]
      }
      frame "---------- Script ----------" {
        # "Template Separator\n(You can make a copy of, or modify, this frame)"
        n124 = call <vilib>:"Add State(s) to Queue__JKI_lib_State_Machine.vi"("State(s) in (\"\")"=w335) -> ("States Out"=w334:string)  [unwired: 14 in]
      }
      frame "Script: Action" {
        n125 = Unbundle By Name(w339) -> ("SystemLink OT"=w336:refnum<class "SystemLinkOutputTerminal.lvclass">, "Script"=w337:string, "scripts manager"=w341:refnum<class "scripts manager.lvclass">)
        n126 = case shown="\"Init\"" w344 {
          tunnel: w343 -> [w347 w354 w359 w363 w369 w372]
          tunnel: [w347 w353 w357 w361 w365 w371] -> w342
          tunnel: w341 -> [w348 _ w358 w362 w368 w373]
          tunnel: [w348 w352 w356 w360 w364 refnum<class "scripts manager.lvclass"> refnum ("scripts manager out")] -> w340
          tunnel: w337 -> [_ _ w355 _ _ _]
          tunnel: w336 -> [_ w349 _ _ _ _]
          frame Default {
          }
          frame "Init" {
            w350 = refnum<class "RT Variables.lvclass"> refnum  # RT Variables
            w351 = refnum<class "scripts manager.lvclass"> refnum  # scripts manager
            n127 = call-dynamic "Instantiate.vi"("scripts manager in"=w351, "Output Terminal"=w349, "RT Variables"=w350, "error in (no error)"=w354) -> ("scripts manager out"=w352:refnum<class "scripts manager.lvclass">, "error out"=w353:errorcluster)  [unwired: 10 in]
          }
          frame "Update" {
            n128 = property class="scripts manager.lvclass"(reference=w358, error in=w359, "properties:Scripts"=w355) -> (reference out=w356:refnum<class "scripts manager.lvclass">, error out=w357:errorcluster)
          }
          frame "Compile" {
            n129 = call-dynamic "Compile Script.vi"("scripts manager in"=w362, "error in (no error)"=w363) -> ("scripts manager out"=w360:refnum<class "scripts manager.lvclass">, "error out"=w361:errorcluster)  [unwired: 12 in]
          }
          frame "Run" {
            n130 = call-dynamic "Compile Script.vi"("scripts manager in"=w368, "error in (no error)"=w369) -> ("scripts manager out"=w367:refnum<class "scripts manager.lvclass">, "error out"=w366:errorcluster)  [unwired: 12 in]
            n131 = call-dynamic "Execute Script.vi"("scripts manager in"=w367, "error in (no error)"=w366) -> ("scripts manager out"=w364:refnum<class "scripts manager.lvclass">, "error out"=w365:errorcluster)  [unwired: 12 in]
          }
          frame "Close" {
            n132 = call-dynamic "Destroy.vi"("scripts manager in"=w373, "error in (no error)"=w372) -> ("error out"=w371:errorcluster)  [unwired: 12 in, 1 out]
          }
        }
        n133 = Bundle By Name(cluster=w339, "scripts manager"=w340) -> (w338:T4)
        n134 = call <vilib>:"Add State(s) to Queue__JKI_lib_State_Machine.vi"("State(s) in (\"\")"=w346) -> ("States Out"=w345:string)  [unwired: 14 in]
      }
      frame "Script: File Operations" {
        n135 = property on="Script Files" class="LstBox (strict)"() -> ("Item Names"=w378:string[], "Value"=w374:i32)  [unwired: 2 in, 2 out]
        n136 = Unbundle By Name(w383) -> ("Config Folder"=w379:path, "Script"=w382:string)
        n137 = Index Array(array=w378, index=w374) -> (element=w381:string)
        n138 = case shown="\"Save Active Script\"" w384 {
          tunnel: w380 -> [w386 w396 w402 w409 w415 w438]
          tunnel: [w386 w393 w400 w407 w419 w433] -> w385
          tunnel: w382 -> [_ _ _ w406 _ _]
          tunnel: w381 -> [_ _ w398 w405 w417 _]
          tunnel: w379 -> [_ w387 w397 w404 w418 _]
          tunnel: w378 -> [_ _ _ _ w413 w434]
          tunnel: [_ _ _ _ w411 w430] -> w375
          tunnel: w374 -> [_ _ _ _ w412 _]
          frame Default {
          }
          frame "List Script File" {
            n139 = List Folder(path=w387, pattern="*.lsl", error in=w396) -> (filenames=w390:string[], error out=w394:errorcluster)  [unwired: 1 in, 2 out]
            n140 = Empty Array?(array=w390) -> (empty?=w391:bool)
            n141 = Select(t=string[] ["main.lsl"], s=w391, f=w390) -> (s? t:f=w389:string[])
            n142 = property on="Script Files" class="LstBox (strict)"(error in=w394, "Item Names"=w389, "Value"=0 ("Files")) -> (error out=w393:errorcluster)  [unwired: 1 in, 1 out]
          }
          frame "Open Active Script" {
            n143 = Build Path(base path=w397, name or relative path=w398) -> (appended path=w403:path)
            n144 = Read from Text File(file (use dialog)=w403, error in=w402) -> (text=w399:string, error out=w401:errorcluster)  [unwired: 2 in, 2 out]
            n145 = property on="Script Editor" class="Str"("Val(Sgnl)"=w399) -> ()  [unwired: 2 in, 2 out]
            n146 = call <vilib>:"Clear Errors.vi"("error in (no error)"=w401) -> ("error out"=w400:errorcluster)  [unwired: 5 in, 1 out]
          }
          frame "Save Active Script" {
            n147 = Build Path(base path=w404, name or relative path=w405) -> (appended path=w410:path)
            n148 = Write to Text File(file (use dialog)=w410, text=w406, error in=w409) -> (error out=w408:errorcluster)  [unwired: 1 in, 2 out]
            n149 = call <vilib>:"Clear Errors.vi"("error in (no error)"=w408) -> ("error out"=w407:errorcluster)  [unwired: 5 in, 1 out]
          }
          frame "Delete Active Script" {
            n150 = Build Path(base path=w418, name or relative path=w417) -> (appended path=w416:path)
            n151 = case shown="Default" w417 {
              tunnel: w416 -> [w427 _]
              tunnel: w415 -> [w428 w429]
              tunnel: [w426 w429] -> w414
              tunnel: w413 -> [w425 _]
              tunnel: w412 -> [w422 _]
              tunnel: ["Script: File Operations >> Open Active Script" _] -> w411
              frame Default {
                n152 = Delete From Array(array=w425, length=1, index=w422) -> (array with subset deleted=w424:string[])  [unwired: 1 out]
                n153 = Delete(path (use dialog)=w427, error in=w428) -> (error out=w426:errorcluster)  [unwired: 3 in, 2 out]
                n154 = property on="Script Files" class="LstBox (strict)"("Item Names"=w424, "Value"=0 ("Script Files")) -> ()  [unwired: 2 in, 2 out]
              }
              frame "main.lsl" {
              }
            }
            n155 = call <vilib>:"Clear Errors.vi"("error in (no error)"=w414) -> ("error out"=w419:errorcluster)  [unwired: 5 in, 1 out]
          }
          frame "New Script File" {
            n156 = call "New Script File"("error in (no error)"=w438) -> ("File Name"=w435:string, "Create"=w436:bool, "error out"=w437:errorcluster)  [unwired: 16 in]
            n157 = Concatenate Strings(w435, ".lsl" ("string")) -> (w432:string)
            n158 = case shown="True" w436 {
              tunnel: w437 -> [w439 w441]
              tunnel: w432 -> [_ w445]
              tunnel: w434 -> [_ w443]
              tunnel: [w439 w441] -> w433
              tunnel: [_ "Script: File Operations >> Open Active Script"] -> w430
              frame False {
              }
              frame True {
                n159 = Build Array (concatenate)(w443, w445) -> (w444:string[])
                n160 = Array Size(array=w443) -> (size(s)=w442:i32)
                n161 = property on="Script Files" class="LstBox (strict)"("Item Names"=w444, "Value"=w442) -> ()  [unwired: 2 in, 2 out]
              }
            }
          }
        }
        n162 = call <vilib>:"Add State(s) to Queue__jki_lib_state_machine.vi"("State(s) in Front (\"\")"=w375, "State(s) in (\"\")"=w376) -> ("States Out"=w377:string)  [unwired: 13 in]
      }
      frame "-------System Link--------" {
      }
      frame "SL: Subscribe" {
        n163 = Unbundle By Name(w451) -> ("topic"=w449:string, "message async"=w453:refnum<class "NI Skyline Message AMQP (Async).lvclass">)
        n164 = call-dynamic "Subscribe.vi"("error in (no error)"=w455, "topic"=w449, "message async"=w453) -> ("error out"=w454:errorcluster, "message async out"=w452:refnum<class "NI Skyline Message AMQP (Async).lvclass">)  [unwired: 7 in]
        n165 = Bundle By Name(cluster=w451, "message async"=w452) -> (w450:T4)
      }
      frame "SL: Unsubscribe & Close" {
        n166 = Unbundle By Name(w463) -> ("topic"=w457:string, "message async"=w464:refnum<class "NI Skyline Message AMQP (Async).lvclass">)
        n167 = call-dynamic "Unsubscribe.vi"("error in (no error)"=w465, "topic"=w457, "message async"=w464) -> ("error out"=w460:errorcluster, "message async out"=w461:refnum<class "NI Skyline Message AMQP (Async).lvclass">)  [unwired: 7 in]
        n168 = call-dynamic "Close.vi"("error in (no error)"=w460, "message async"=w461) -> ("error out"=w459:errorcluster)  [unwired: 9 in]
        n169 = Bundle By Name(cluster=w463, "message async"=refnum<class "NI Skyline Message AMQP (Async).lvclass"> refnum) -> (w462:T4)
      }
    }
  }
